vi "State Machine Starter Helper.vi"   [LabVIEW 2019, in "State Machine API.lvlib"]
uses:
  State Machine API.lvlib
  Actions Template.vit
  Guards Template.vit
  70c83eff-f1e3-48ad-9bec-1669ecfcf6fa.vi
  3b5fd4a9-f72b-422d-98a2-4c48f226a3c8.vi
types:
  T1 = map{enum16{"state 1"}, map{enum16{"event 1"}, cluster{"State Type":enum16{"state 1"}, "Action Type":enum16{"action 1"}, bool, "Guard Type":enum16{"guard 1"}, bool}[]}}
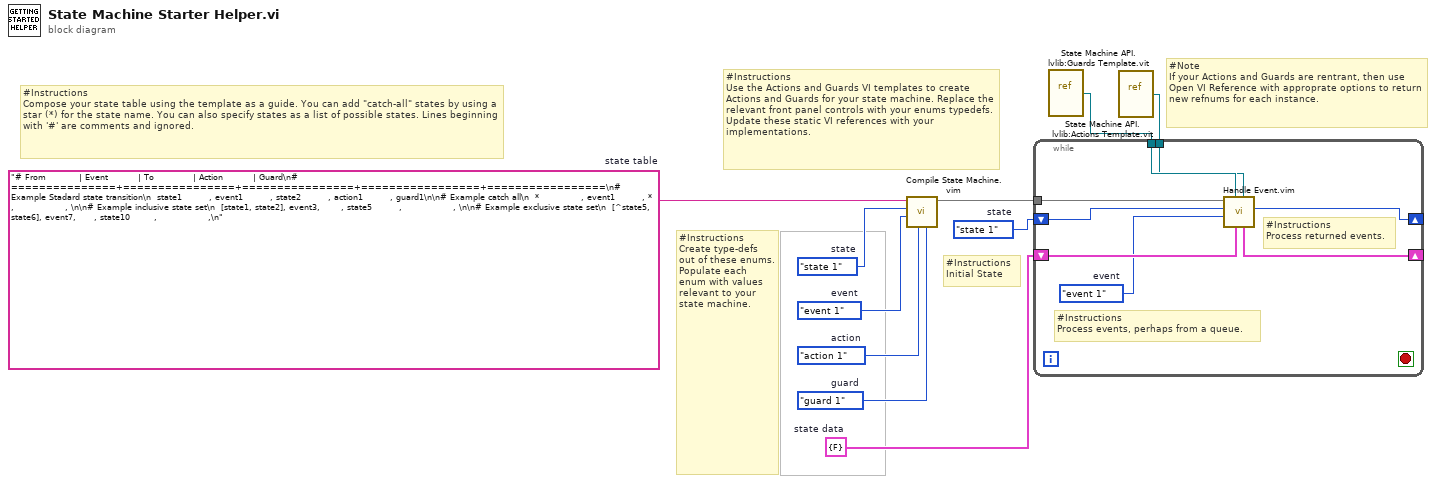
[diagram p0: block diagram]
diagram:
  w1 = enum16{"state 1"}."state 1"  # state
  w2 = enum16{"guard 1"}."guard 1"  # guard
  w3 = enum16{"action 1"}."action 1"  # action
  w4 = enum16{"event 1"}."event 1"  # event
  w5 = enum16{"state 1"}."state 1"  # state
  w6 = cluster{"value":bool} {"value"=FALSE}  # state data
  w10 = "# From           | Event          | To             | Action          | Guard\n# ===============+================+================+=================+=================\n# Example Stadard state transition\n  state1         , event1         , state2         , action1         , guard1\n\n# Example catch all\n  *              , event1         , *              ,                 , \n\n# Example inclusive state set\n  [state1, state2], event3,       , state5         ,                 , \n\n# Example exclusive state set\n  [^state5, state6], event7,      , state10        ,                 ,\n"  # state table
  # "#Note\nIf your Actions and Guards are rentrant, then use Open VI Reference with approprate options to return new refnums for each instance."
  # "#Instructions\nInitial State"
  # "#Instructions\nCompose your state table using the template as a guide. You can add \"catch-all\" states by using a star (*) for the state name. You can also specify states as a list of possible states. Lines beginning with '#' are comments and ignored."
  # "#Instructions\nUse the Actions and Guards VI templates to create Actions and Guards for your state machine. Replace the relevant front panel controls with your enums typedefs. Update these static VI references with your implementations."
  # "#Instructions\nCreate type-defs out of these enums. Populate each enum with values relevant to your state machine."
  n1 = call "Compile State Machine.vim"("Guard Type"=w2, "Action Type"=w3, "Event Type"=w4, "State Type"=w5, "state machine definition"=w10) -> ("map"=w9:T1)  [unwired: 5 in, 1 out]
  n2 = vi-ref "State Machine API.lvlib:Guards Template.vit"() -> (w7:refnum<vi>)
  n3 = vi-ref "State Machine API.lvlib:Actions Template.vit"() -> (w8:refnum<vi>)
  n4 = while {
    tunnel: w9 -> [w16]
    shift-right: [w17] -> _
    shift-left: w1 -> [w13]
    tunnel: w8 -> [w14]
    tunnel: w7 -> [w15]
    shift-right: [w18] -> _
    shift-left: w6 -> [w12]
    stop <- _ stop-if-true
    w11 = enum16{"event 1"}."event 1"  # event
    # "#Instructions\nProcess returned events."
    # "#Instructions\nProcess events, perhaps from a queue."
    n5 = call "Handle Event.vim"("actions"=w14, "state data in"=w12, "guards"=w15, "event"=w11, "state in"=w13, "compiled state machine"=w16) -> ("state out"=w17:enum16{"state 1"}, "state data out"=w18:cluster{"value":bool})  [unwired: 2 in, 2 out]
  }
